vi "y1y2 (子VI)备份2.vi"(0 "Image Pixels (U8)输入":u8[][](array[numeric])) -> (4 "平均left":cluster{i32, i32}[](array[cluster]), 6 "平均left 2":cluster{i32, i32}[](array[cluster]), 7 "left":cluster{i32, i32}[](graph), 8 "out left point":cluster{i32, i32}[](array[cluster]), 9 "right":cluster{i32, i32}[](graph), 10 "out right point 2":cluster{i32, i32}[](array[cluster]))   [LabVIEW 2014]
uses:
  <vilib>/Analysis/baseanly.llb/Mean (DBL).vi
  <vilib>/Analysis/NI_AALBase.lvlib
panel:
  out "x2max":cluster{i32, i32}
  out "x2min":cluster{i32, i32}
  out "y2max":cluster{i32, i32}
  out "y2min":cluster{i32, i32}
  out "y1min":cluster{i32, i32}
  out "y1max":cluster{i32, i32}
  out "x1min":cluster{i32, i32}
  out "x1max":cluster{i32, i32}
  # "3"
  # "4"
  # "x"
  # "1"
  # "2"
  # "y"
  # "x"
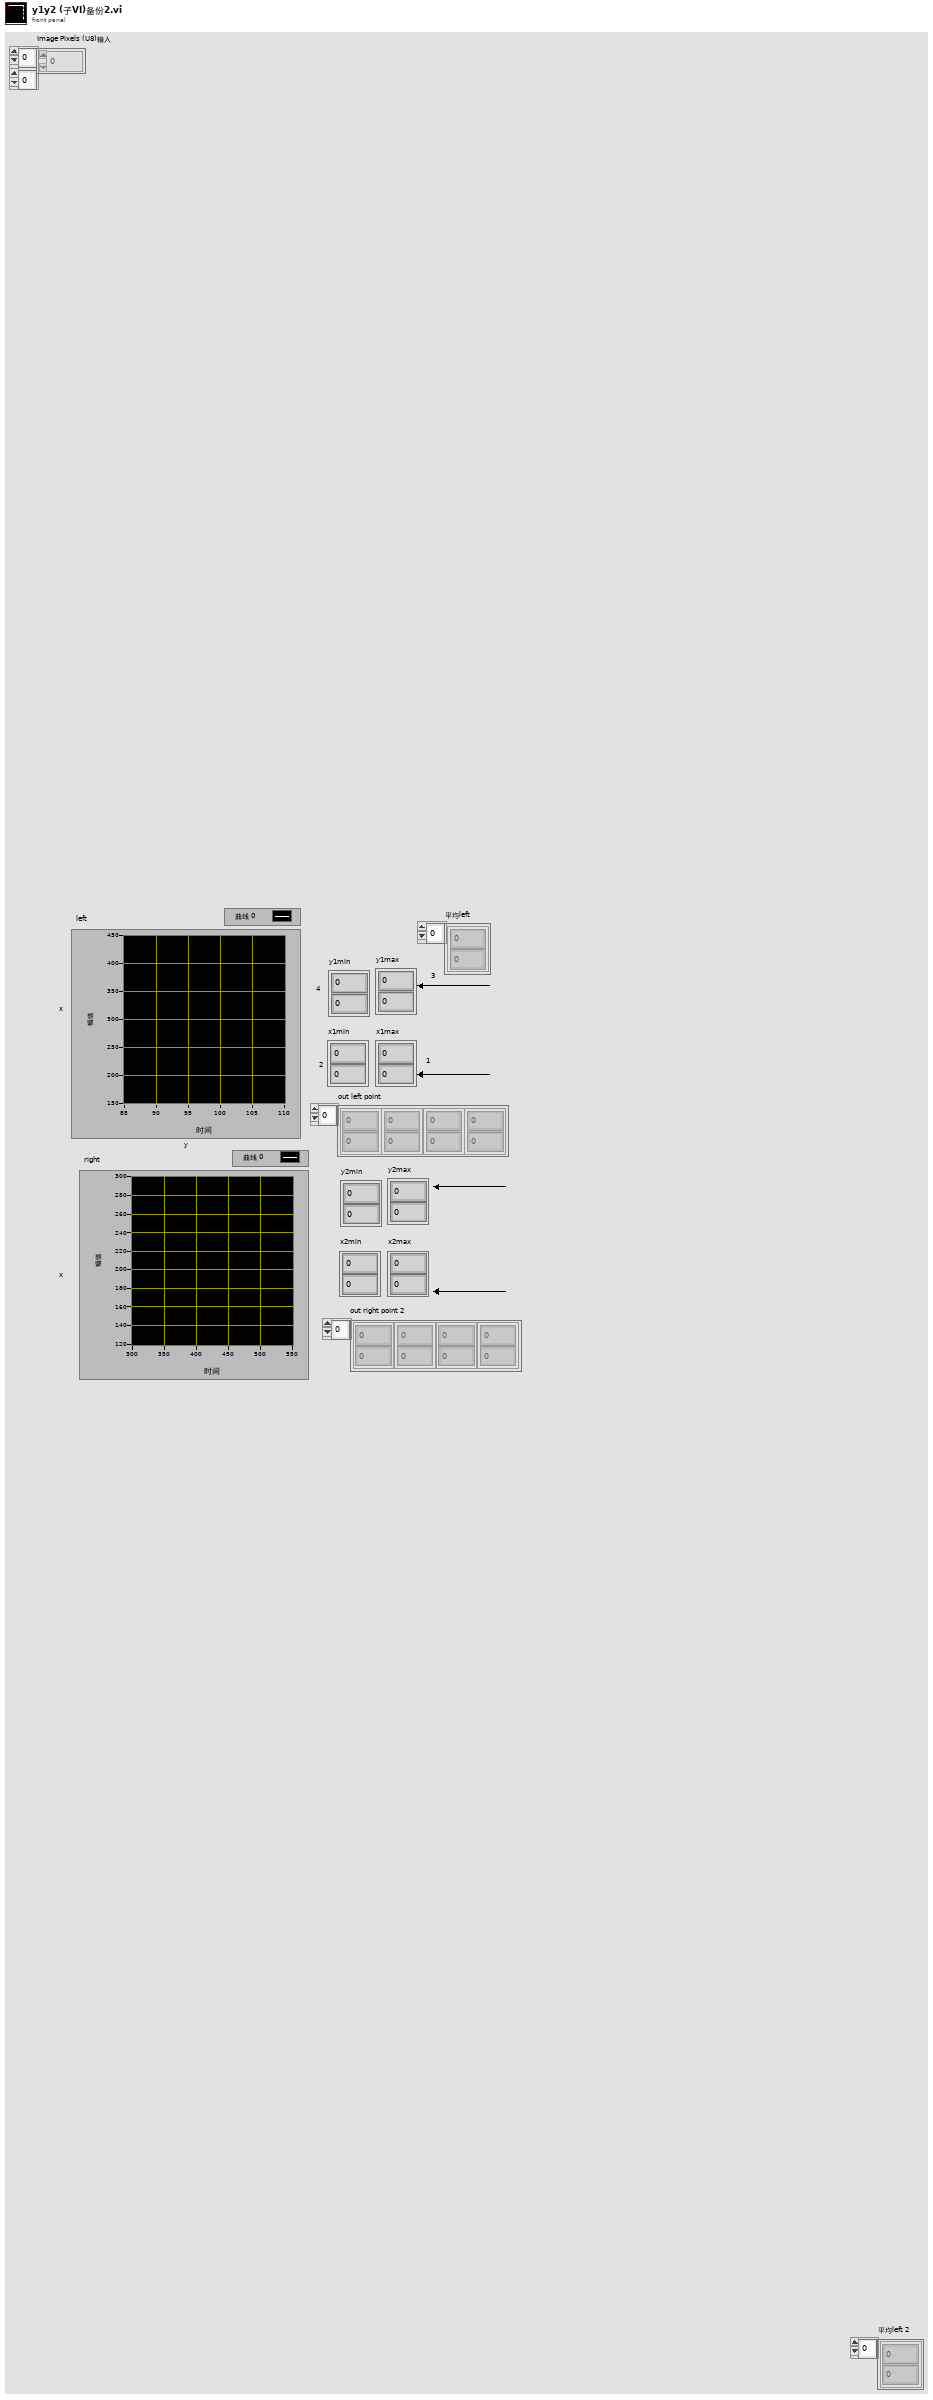
[diagram p1: front panel]
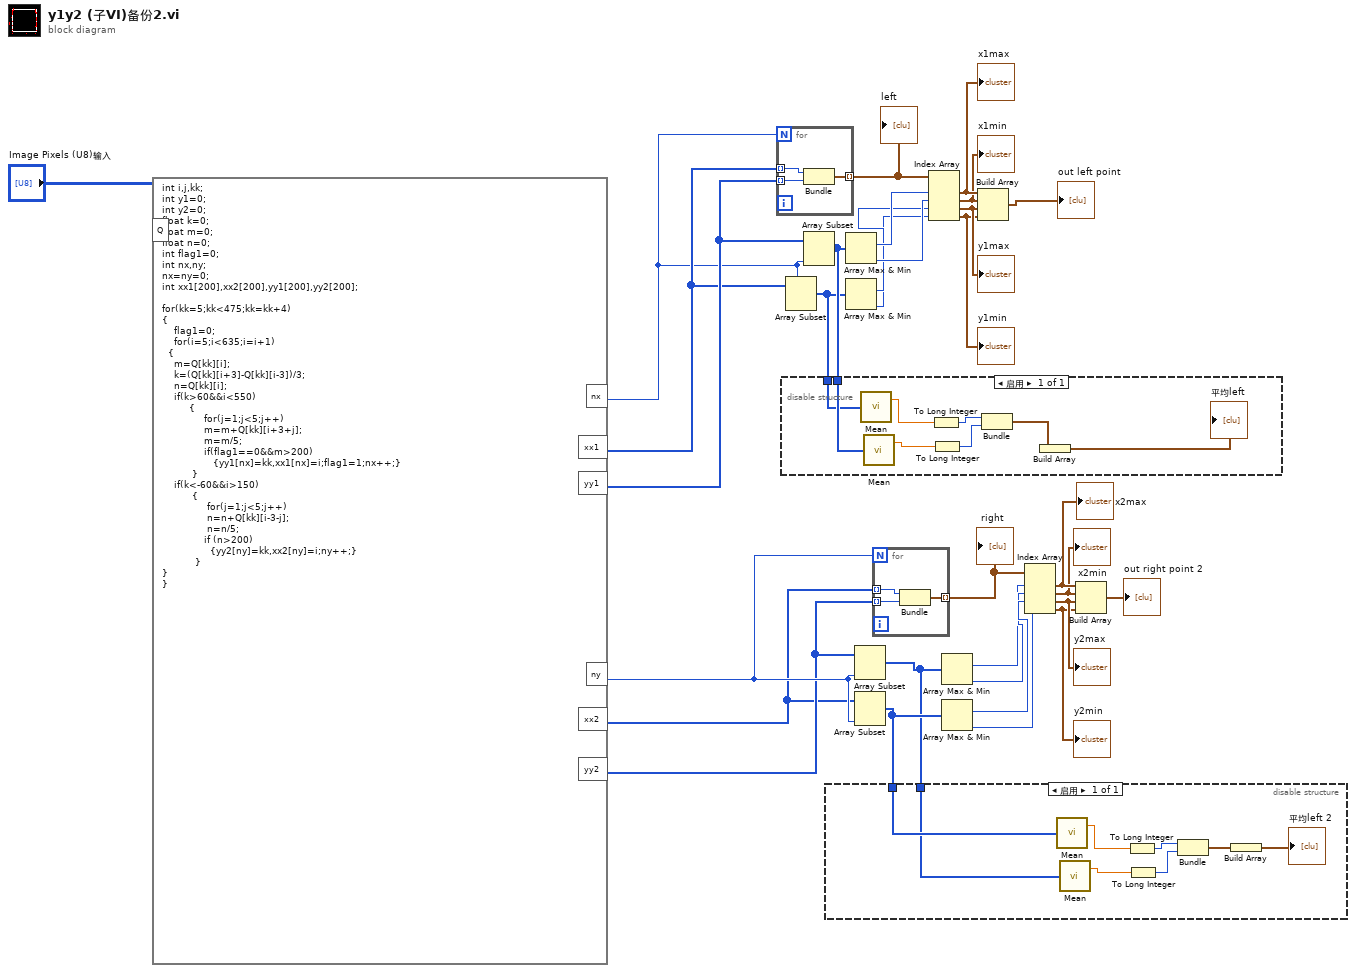
[diagram p0: block diagram]
diagram:
  n1 = formula code="int i,j,kk;\nint y1=0;\nint y2=0;\nfloat k=0;\nfloat m=0;\nfloat n=0;\nint flag1=0;\nint nx,ny;\nnx=ny=0;\nint xx1[200],xx2[200],yy1[200],yy2[200];\n\nfor(kk=5;kk<475;kk=kk+4)\n{\n    flag1=0;\n    for(i=5;i<635;i=i+1)\n  {\n    m=Q[kk][i];\n    k=(Q[kk][i+3]-Q[kk][i-3])/3;\n    n=Q[kk][i];\n    if(k>60&&i<550)\n         {   \n              for(j=1;j<5;j++)\n              m=m+Q[kk][i+3+j];\n              m=m/5;\n              if(flag1==0&&m>200)\n                 {yy1[nx]=kk,xx1[nx]=i;flag1=1;nx++;}\n          }\n    if(k<-60&&i>150)\n          {                   \n               for(j=1;j<5;j++)\n               n=n+Q[kk][i-3-j];\n               n=n/5;\n              if (n>200)\n                {yy2[ny]=kk,xx2[ny]=i;ny++;}\n           }\n}\n}"("Q"="Image Pixels (U8)输入") -> ("xx1"=w25:i32[], "yy1"=w26:i32[], "nx"=w24:i32, "xx2"=w16:i32[], "yy2"=w17:i32[], "ny"=w18:i32)
  n2 = for {
    N: w24 -> [_]
    tunnel: w25 -> [w34] mode=indexing
    tunnel: w26 -> [w33] mode=indexing
    tunnel: [w32] -> w31 mode=indexing
    n3 = Bundle(w34, w33) -> (w32:cluster{i32, i32})  [unwired: 1 in]
  }
  "left" <- w31
  n4 = Array Subset(array=w25, length=w24) -> (w4:i32[])  [unwired: 1 in]
  n5 = Array Subset(array=w26, length=w24) -> (w5:i32[])  [unwired: 1 in]
  n6 = disable-structure shown="启用" {
    disable-tunnel: w5 -> [w42]
    disable-tunnel: w4 -> [w41]
    frame Enabled {
      n7 = call-poly <vilib>:"Mean.vi"("X"=w41) -> ("mean"=w39:dbl)  [unwired: 1 out]
      n8 = call-poly <vilib>:"Mean.vi"("X"=w42) -> ("mean"=w40:dbl)  [unwired: 1 out]
      n9 = To Long Integer(number=w39) -> (32bit integer=w38:i32)
      n10 = To Long Integer(number=w40) -> (32bit integer=w37:i32)
      n11 = Bundle(w38, w37) -> (w36:cluster{i32, i32})  [unwired: 1 in]
      n12 = Build Array(w36) -> (→"平均left":cluster{i32, i32}[])
    }
  }
  n13 = Array Max & Min(array=w5) -> (max index (indices)=w30:i32, min index (indices)=w29:i32)  [unwired: 2 out]
  n14 = Array Max & Min(array=w4) -> (max index (indices)=w28:i32, min index (indices)=w27:i32)  [unwired: 2 out]
  n15 = Array Subset(array=w17, length=w18) -> (w1:i32[])  [unwired: 1 in]
  n16 = Array Subset(array=w16, length=w18) -> (w2:i32[])  [unwired: 1 in]
  n17 = disable-structure shown="启用" {
    disable-tunnel: w2 -> [w44]
    disable-tunnel: w1 -> [w43]
    frame Enabled {
      n18 = call-poly <vilib>:"Mean.vi"("X"=w44) -> ("mean"=w49:dbl)  [unwired: 1 out]
      n19 = call-poly <vilib>:"Mean.vi"("X"=w43) -> ("mean"=w50:dbl)  [unwired: 1 out]
      n20 = To Long Integer(number=w49) -> (32bit integer=w48:i32)
      n21 = To Long Integer(number=w50) -> (32bit integer=w47:i32)
      n22 = Bundle(w48, w47) -> (w46:cluster{i32, i32})  [unwired: 1 in]
      n23 = Build Array(w46) -> (→"平均left 2":cluster{i32, i32}[])
    }
  }
  n24 = for {
    N: w18 -> [_]
    tunnel: w16 -> [w53] mode=indexing
    tunnel: w17 -> [w52] mode=indexing
    tunnel: [w51] -> w19 mode=indexing
    n25 = Bundle(w53, w52) -> (w51:cluster{i32, i32})  [unwired: 1 in]
  }
  "right" <- w19
  n26 = Index Array(array=w31, index #1=w30, index #2=w29, index #3=w28, index #4=w27) -> (element #1=w14:cluster{i32, i32}, element #2=w13:cluster{i32, i32}, element #3=w12:cluster{i32, i32}, element #4=w11:cluster{i32, i32})
  "x1max" <- w14
  "x1min" <- w13
  "y1max" <- w12
  "y1min" <- w11
  n27 = Array Max & Min(array=w1) -> (max index (indices)=w20:i32, min index (indices)=w21:i32)  [unwired: 2 out]
  n28 = Array Max & Min(array=w2) -> (max index (indices)=w22:i32, min index (indices)=w23:i32)  [unwired: 2 out]
  n29 = Build Array(w14, w13, w12, w11) -> (→"out left point":cluster{i32, i32}[])
  n30 = Index Array(array=w19, index #1=w20, index #2=w21, index #3=w22, index #4=w23) -> (element #1=w9:cluster{i32, i32}, element #2=w8:cluster{i32, i32}, element #3=w7:cluster{i32, i32}, element #4=w6:cluster{i32, i32})
  "x2max" <- w9
  "x2min" <- w8
  "y2max" <- w7
  "y2min" <- w6
  n31 = Build Array(w9, w8, w7, w6) -> (→"out right point 2":cluster{i32, i32}[])
